vi "Start Measurements.vi"(6 "Reply to":refnum<class "Result Reply Msg.lvclass">, 7 "Objects enqueuers":refnum<class "Message Enqueuer.lvclass">[](array[class]), 8 "error in (no error)":errorcluster, 10 "Objects":string[](array[string]), 11 "Monitor Controller in":refnum<class "Monitor Controller.lvclass">) -> (0 "error out":errorcluster, 3 "Monitor Controller out":refnum<class "Monitor Controller.lvclass">)   [LabVIEW 2016, in "Monitor Controller.lvclass"]
uses:
  Monitor Controller.lvclass
  C:/github/LabActor/Worker/Worker.lvclass
  C:/github/LabActor/Controllers/Process Controller/Process Controller.lvclass
  Template Module Messages/Result Reply Msg/Result Reply Msg.lvclass
  <vilib>/ActorFramework/Message Enqueuer/Message Enqueuer.lvclass
  Worker/Worker.lvclass/Worker.ctl
  Monitor Controller.lvclass/Monitor Controller.ctl
  Process Controller/Process Controller.lvclass/Process Controller.ctl
  Worker/Write Cycle period.vi
  Process Controller/Write Repeat times.vi
  Template Module/Read State.vi
  Read Monitor controller configuration.vi
  Process Controller/Process Controller.lvclass
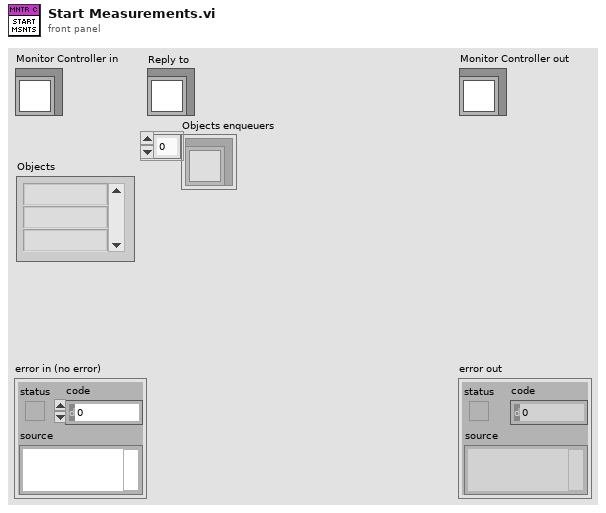
[diagram p1: front panel]
types:
  T1 = typedef "Worker State.ctl" = enum16{"Idle", "Starting", "Working", "Stopping"}
  T2 = typedef "Monitor Controller Configuration.ctl" = cluster{"Update period":dbl, "Repeat times":i32, "Open plot":bool, "File defragment period":dbl}
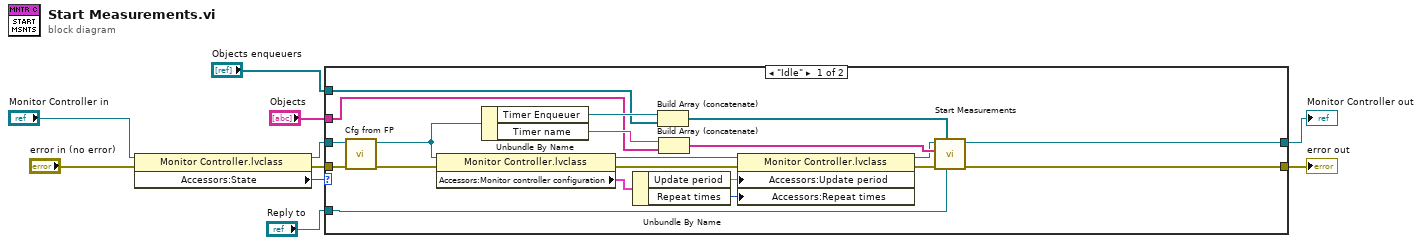
[diagram p0: block diagram]
diagram:
  n1 = property class="Monitor Controller.lvclass"(reference="Monitor Controller in", error in="error in (no error)") -> (reference out=w5:refnum<class "Monitor Controller.lvclass">, error out=w3:errorcluster, "Accessors:State"=w1:T1)
  n2 = case shown="\"Idle\"" w1 {
    tunnel: "Reply to" -> [w30 _]
    tunnel: "Objects enqueuers" -> [w28 _]
    tunnel: "Objects" -> [w26 _]
    tunnel: [w22 w31] -> w6
    tunnel: w5 -> [w14 w32]
    tunnel: w3 -> [w13 w31]
    tunnel: [w23 w32] -> w2
    frame "Idle" {
      n3 = call-dynamic "Cfg from FP.vi"("error in (no error)"=w13, "Measure Object in"=w14) -> ("error out"=w12:errorcluster, "Measure Object out"=w11:refnum<class "Monitor Controller.lvclass">)  [unwired: 8 in]
      n4 = property class="Monitor Controller.lvclass"(reference=w11, error in=w12) -> (reference out=w20:refnum<class "Monitor Controller.lvclass">, error out=w16:errorcluster, "Accessors:Monitor controller configuration"=w19:T2)
      n5 = Unbundle By Name(w11) -> ("Timer Enqueuer"=w29:refnum<class "Message Enqueuer.lvclass">, "Timer name"=w27:string)
      n6 = Unbundle By Name(w19) -> ("Update period"=w18:dbl, "Repeat times"=w15:i32)
      n7 = Build Array (concatenate)(w29, w28) -> (w25:refnum<class "Message Enqueuer.lvclass">[])
      n8 = Build Array (concatenate)(w27, w26) -> (w24:string[])
      n9 = property class="Monitor Controller.lvclass"(reference=w20, error in=w16, "Accessors:Update period"=w18, "Accessors:Repeat times"=w15) -> (reference out=w21:refnum<class "Monitor Controller.lvclass">, error out=w17:errorcluster)
      n10 = call-parent "Start Measurements.vi"("Reply to"=w30, "Objects enqueuers"=w25, "error in (no error)"=w17, "Objects"=w24, "Measure Controller in"=w21) -> ("error out"=w22:errorcluster, "Measure Controller out"=w23:refnum<class "Monitor Controller.lvclass">)  [unwired: 5 in]
    }
    frame "Working", Default {
    }
  }
  "error out" <- w6
  "Monitor Controller out" <- w2
